vi "Initialize Attributes.vi"(8 "error in (no error)":errorcluster, 10 "Attribute Data":variant, 11 "CS++TestMotor in":refnum<class "CS++TestMotor.lvclass">) -> (0 "error out":errorcluster, 2 "Found?":bool, 3 "CS++TestMotor out":refnum<class "CS++TestMotor.lvclass">)   [LabVIEW 2015, in "CS++TestMotor.lvlib" / "CS++TestMotor.lvclass"]
doc: "Initialize object attribute.\n\nUnique resources should be allocated elsewhere!"
uses:
  CS++TestMotor.lvclass
  CS++TestMotor.lvclass/CS++TestMotor.ctl
  CSPP_Core/Actors/CS++BaseActor/CS++BaseActor.lvclass/CS++BaseActor.ctl
  CSPP_Core/Actors/CS++BaseActor/CS++BaseActor.lvclass
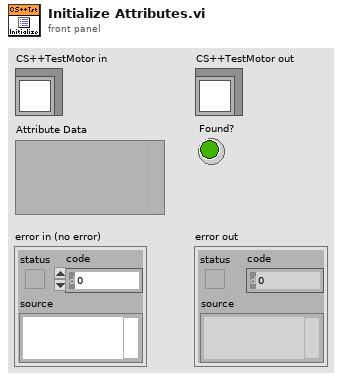
[diagram p1: front panel]
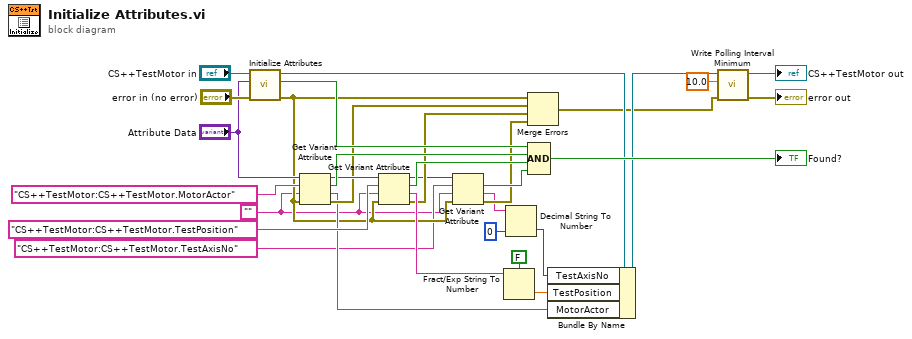
[diagram p0: block diagram]
diagram:
  w8 = ""
  n1 = call-parent "Initialize Attributes.vi"("error in (no error)"="error in (no error)", "Attribute Data"="Attribute Data", "CS++BaseActor in"="CS++TestMotor in") -> ("error out"=w14:errorcluster, "Found?"=w21:bool, "CS++BaseActor out"=w17:refnum<class "CS++TestMotor.lvclass">)  [unwired: 6 in]
  n2 = Get Variant Attribute(Variant="Attribute Data", name="CS++TestMotor:CS++TestMotor.MotorActor", default value (empty Variant)=w8, error in=w14) -> (duplicate Variant=w26:variant, found=w27:bool, value=w15:string, error out=w19:errorcluster)
  n3 = Get Variant Attribute(Variant=w26, name="CS++TestMotor:CS++TestMotor.TestPosition", default value (empty Variant)=w8, error in=w14) -> (duplicate Variant=w13:variant, found=w22:bool, value=w24:string, error out=w18:errorcluster)
  n4 = Get Variant Attribute(Variant=w13, name="CS++TestMotor:CS++TestMotor.TestAxisNo", default value (empty Variant)=w8, error in=w14) -> (found=w11:bool, value=w9:string, error out=w10:errorcluster)  [unwired: 1 out]
  n5 = Fract/Exp String To Number(use system decimal point (T)=FALSE, string=w24) -> (number=w16:dbl)  [unwired: 2 in, 1 out]
  n6 = Decimal String To Number(string=w9, default (0L)=u8 0 ("default (0 I32)")) -> (number=w6:u8)  [unwired: 1 in, 1 out]
  n7 = Merge Errors(w14, w19, w18, w10) -> (w3:errorcluster)
  n8 = Compound Arithmetic op=AND(w21, w27, w22, w11) -> (→"Found?":bool)
  n9 = Bundle By Name(cluster=w17, "TestAxisNo"=w6, "TestPosition"=w16, "MotorActor"=w15) -> (w5:refnum<class "CS++TestMotor.lvclass">)
  n10 = call "Write Polling Interval Minimum.vi"("error in (no error)"=w3, "Polling Interval Minimum"=dbl[unit] 10.0, "CS++BaseActor in"=w5) -> ("error out"=→"error out":errorcluster, "CS++BaseActor out"=→"CS++TestMotor out":refnum<class "CS++TestMotor.lvclass">)  [unwired: 7 in]
